vi "SNReport.vi"(6 "SN":string="1", 7 "Slot":T1, 8 "error in (no error)":errorcluster caption="错误输入（无错误）", 9 "字符串":string="测试报告\\条码\\", 10 "列首字符串":string[](array[string])=["ICCID", "IMSI", "AKEY", "ESN", "EVDO账号", "EVDO密码", "MDN", "MEID", "T-BOX-SN", "时间"]) -> (0 "error out":errorcluster caption="错误输出")   [LabVIEW 2013]
uses:
  SystemCode/SysControl/Slot.ctl
  <vilib>/addons/_office/_wordsub.llb/font.ctl
  <vilib>/Utility/NIReport.llb/NI_report.lvclass
  GlobalValue.vi
  <vilib>/addons/_office/excel.llb/Excel Easy Table (str).vi
  <vilib>/Utility/NIReport.llb/Append Text Table to Report (wrap).vi
  <vilib>/addons/_office/NI_ReportGenerationToolkit.lvlib
  <vilib>/Utility/NIReport.llb/Excel/NI_Excel.lvclass
panel:
  out "数组":string[][](array[string])
  in  "TestItem":string="BCM"
  # "产品名称\t序列号\t测试时间\t测试项目\t初始条件\t测试动作\t评价标准\t步骤 测试结果\t测试条件设置"
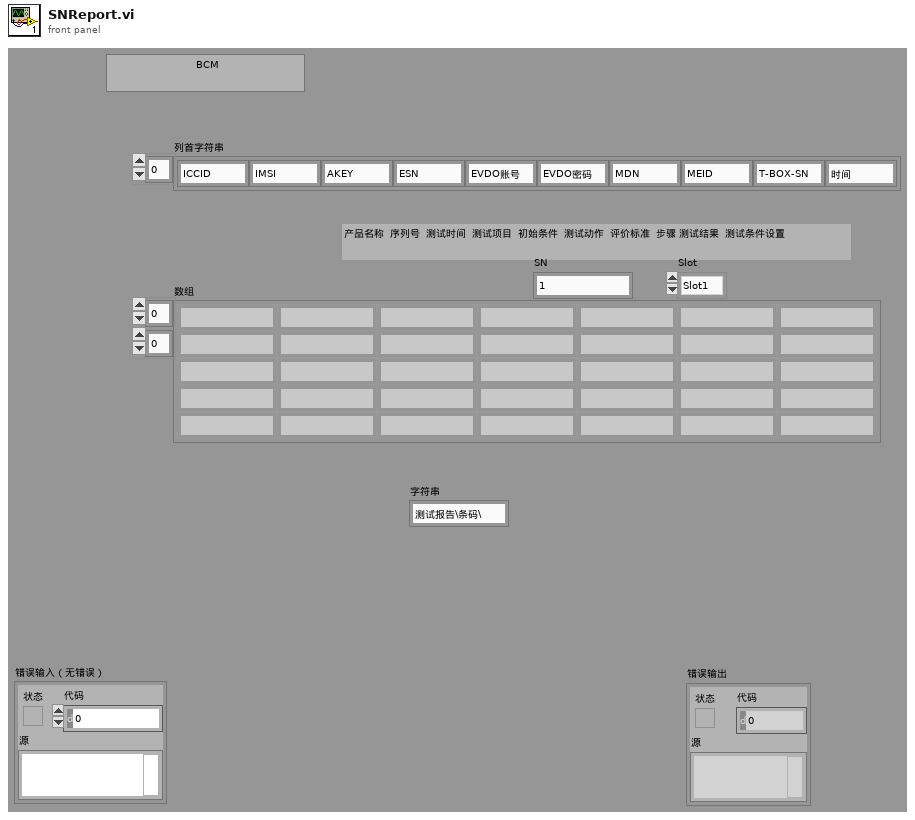
[diagram p1: front panel]
types:
  T1 = typedef "Slot.ctl" = enum16{"Slot1", "Slot2", "Slot3", "Slot4"}
  T2 = enum16{"open", "replace", "create", "open or create", "replace or create", "replace or create with confirmation"}
  T3 = typedef "font.ctl" = cluster{"font name":string, "font size":dbl, "bold":u16, "italic":u16, "underline":u16, "strike through":u16, "font color":u32}
  T4 = enum16{"maximized", "minimized", "normal", "no change"}
  T5 = enum16{"Standard Report", "HTML", "Word", "Excel"}
  T6 = cluster{"on/off":bool, "weight":i32, "color":u32}
  T7 = cluster{"position (Excel)":cluster{"row":i32, "column":i32}, "name (Excel)":string, "bookmark (Word)":string}
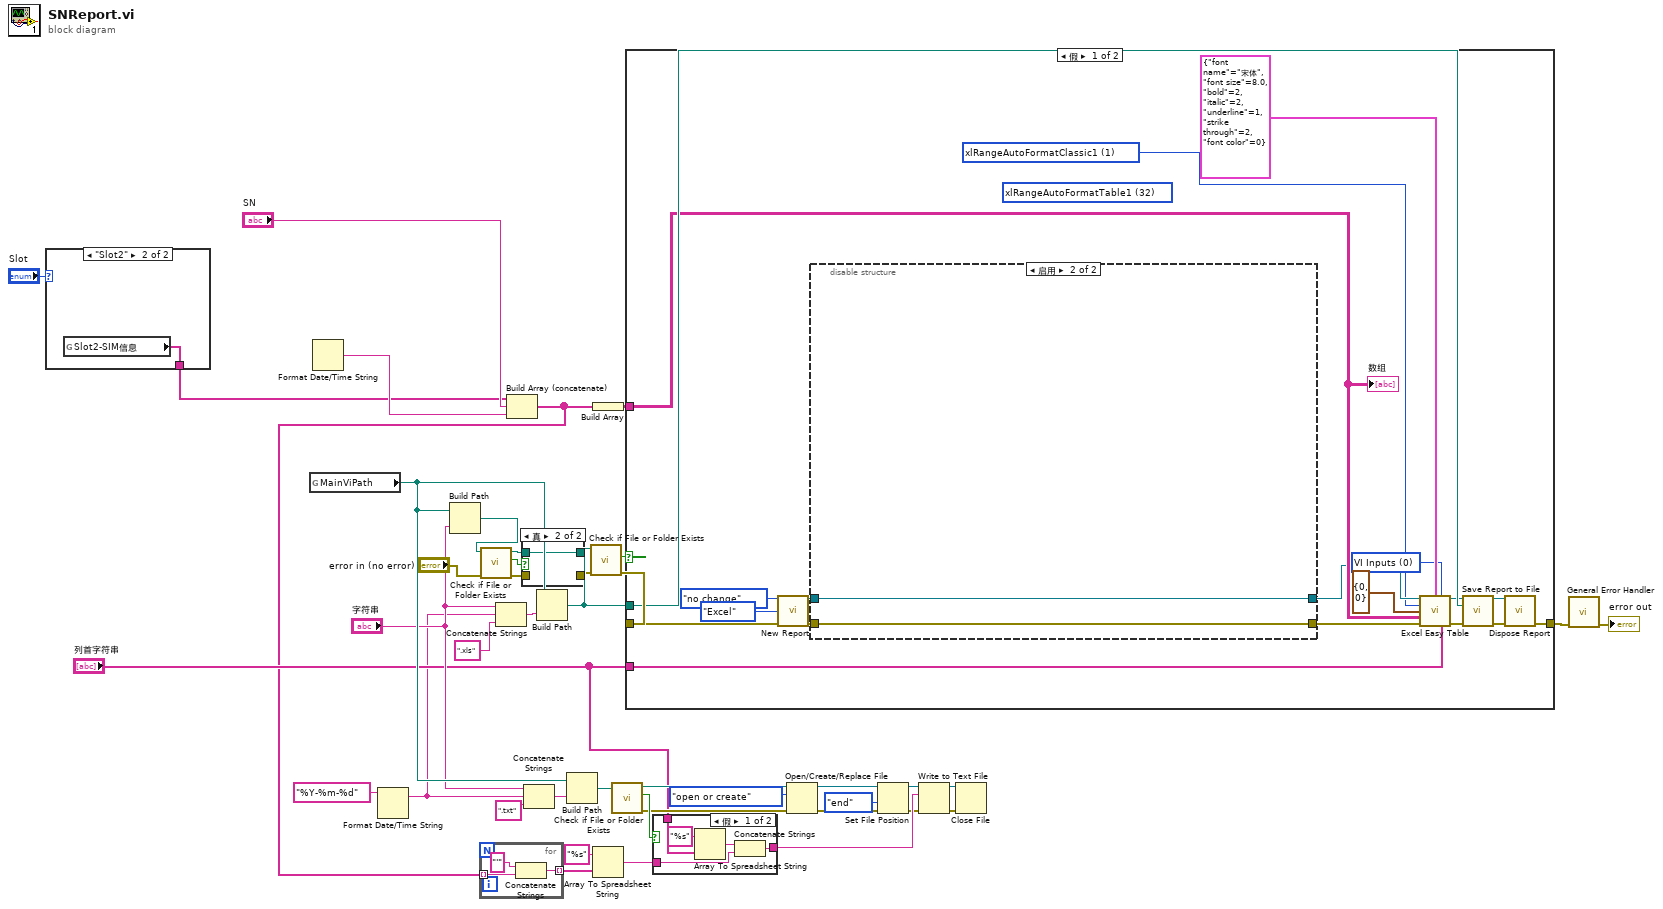
[diagram p0: block diagram]
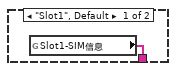
[diagram p3: hidden frame]
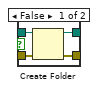
[diagram p4: hidden frame]
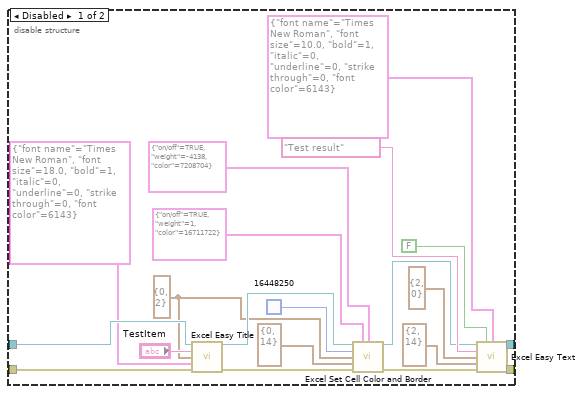
[diagram p5: hidden frame]
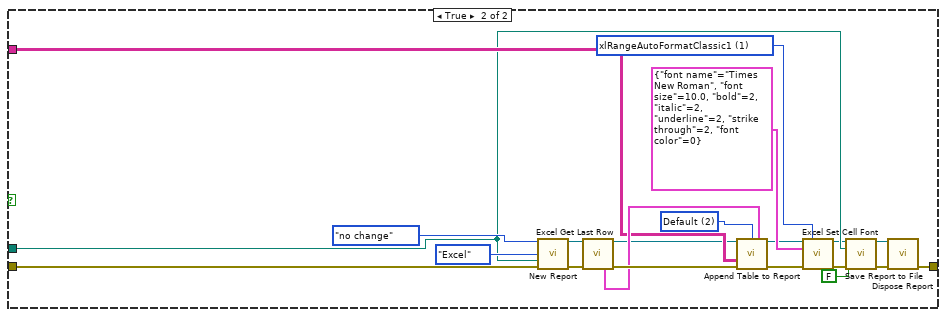
[diagram p6: hidden frame]
diagram:
  n1 = case shown="\"Slot2\"" "Slot" {
    tunnel: [w43 w44] -> w4
    frame "Slot1", Default {
      n2 = global read "GlobalValue.vi" "Slot1-SIM信息"() -> (w43:string[])
    }
    frame "Slot2" {
      n3 = global read "GlobalValue.vi" "Slot2-SIM信息"() -> (w44:string[])
    }
  }
  n4 = global read "GlobalValue.vi" "MainViPath"() -> (w7:path)
  n5 = Format Date/Time String() -> (date/time string=w26:string)  [unwired: 3 in]
  n6 = Format Date/Time String(time format string (%c)="%Y-%m-%d" ("时间格式字符串(%c)")) -> (date/time string=w1:string)  [unwired: 2 in]
  n7 = Build Path(base path=w7, name or relative path="字符串") -> (appended path=w33:path)
  n8 = call <vilib>:"Check if File or Folder Exists.vi"("error in (no error)"="error in (no error)", "path"=w33) -> ("error out"=w35:errorcluster, "file or folder exists?"=w34:bool, "dup path"=w36:path)  [unwired: 7 out]
  n9 = Concatenate Strings("字符串", w1, ".xls" ("连接的字符串")) -> (w38:string)
  n10 = Build Array (concatenate)(w4, "SN", w26) -> (w3:string[])
  n11 = for {
    tunnel: w3 -> [w47] mode=indexing
    tunnel: [w45] -> w20 mode=indexing
    n12 = Concatenate Strings("'" ("字符串"), w47) -> (w45:string)
  }
  n13 = case shown="真" w34 {
    tunnel: w36 -> [w51 w52]
    tunnel: [w50 _] -> w31
    tunnel: w35 -> [w49 _]
    tunnel: [w48 w52] -> _
    frame False {
      n14 = Create Folder(path (use dialog)=w51, error in=w49) -> (created path=w48:path, error out=w50:errorcluster)  [unwired: 2 out]
    }
    frame True {
    }
  }
  n15 = Concatenate Strings("字符串", w1, ".txt" ("连接的字符串")) -> (w17:string)
  n16 = Build Path(base path=w7, name or relative path=w38) -> (appended path=w42:path)
  n17 = Build Path(base path=w7, name or relative path=w17) -> (appended path=w16:path)
  n18 = call <vilib>:"Check if File or Folder Exists.vi"("error in (no error)"=w31, "path"=w42) -> ("error out"=w40:errorcluster, "file or folder exists?"=w39:bool)  [unwired: 8 out]
  n19 = Build Array(w3) -> (w28:string[][])
  n20 = Array To Spreadsheet String(array=w20, 3:"%s" ("格式字符串")) -> (spreadsheet string=w14:string)  [unwired: 1 in]
  n21 = call <vilib>:"Check if File or Folder Exists.vi"("path"=w16) -> ("error out"=w11:errorcluster, "file or folder exists?"=w15:bool, "dup path"=w12:path)  [unwired: 1 in, 7 out]
  n22 = case shown="假" w39 {
    tunnel: w40 -> [w70 w113]
    tunnel: w42 -> [w62 w106]
    tunnel: [w65 w112] -> w41
    tunnel: w28 -> [w61 w108]
    tunnel: "列首字符串" -> [w53 _]
    frame False {
      w54 = u16 0 items=["VI Inputs", "Font Dialog Box"] ("font settings source")
      w56 = 1 items=["xlRangeAutoFormat3DEffects1"=13, "xlRangeAutoFormat3DEffects2"=14, "xlRangeAutoFormatAccounting1"=4, "xlRangeAutoFormatAccounting2"=5, "xlRangeAutoFormatAccounting3"=6, "xlRangeAutoFormatAccounting4"=17, "xlRangeAutoFormatClassic1"=1, "xlRangeAutoFormatClassic2"=2, "xlRangeAutoFormatClassic3"=3, "xlRangeAutoFormatColor1"=7, "xlRangeAutoFormatColor2"=8, "xlRangeAutoFormatColor3"=9, "xlRangeAutoFormatList1"=10, "xlRangeAutoFormatList2"=11, "xlRangeAutoFormatList3"=12, "xlRangeAutoFormatLocalFormat1"=15, "xlRangeAutoFormatLocalFormat2"=16, "xlRangeAutoFormatLocalFormat3"=19, "xlRangeAutoFormatLocalFormat4"=20, "xlRangeAutoFormatReport1"=21, "xlRangeAutoFormatReport2"=22, "xlRangeAutoFormatReport3"=23, "xlRangeAutoFormatReport4"=24, "xlRangeAutoFormatReport5"=25, "xlRangeAutoFormatReport6"=26, "xlRangeAutoFormatReport7"=27, "xlRangeAutoFormatReport8"=28, "xlRangeAutoFormatReport9"=29, "xlRangeAutoFormatReport10"=30, "xlRangeAutoFormatClassicPivotTable"=31, "xlRangeAutoFormatTable1"=32, "xlRangeAutoFormatTable2"=33, "xlRangeAutoFormatTable3"=34, "xlRangeAutoFormatTable4"=35, "xlRangeAutoFormatTable5"=36, "xlRangeAutoFormatTable6"=37, "xlRangeAutoFormatTable7"=38, "xlRangeAutoFormatTable8"=39, "xlRangeAutoFormatTable9"=40, "xlRangeAutoFormatTable10"=41, "xlRangeAutoFormatPTNone"=42, "xlRangeAutoFormatNone"=-4142, "xlRangeAutoFormatSimple"=-4154] ("auto format")
      (unwired) 32 items=["xlRangeAutoFormat3DEffects1"=13, "xlRangeAutoFormat3DEffects2"=14, "xlRangeAutoFormatAccounting1"=4, "xlRangeAutoFormatAccounting2"=5, "xlRangeAutoFormatAccounting3"=6, "xlRangeAutoFormatAccounting4"=17, "xlRangeAutoFormatClassic1"=1, "xlRangeAutoFormatClassic2"=2, "xlRangeAutoFormatClassic3"=3, "xlRangeAutoFormatColor1"=7, "xlRangeAutoFormatColor2"=8, "xlRangeAutoFormatColor3"=9, "xlRangeAutoFormatList1"=10, "xlRangeAutoFormatList2"=11, "xlRangeAutoFormatList3"=12, "xlRangeAutoFormatLocalFormat1"=15, "xlRangeAutoFormatLocalFormat2"=16, "xlRangeAutoFormatLocalFormat3"=19, "xlRangeAutoFormatLocalFormat4"=20, "xlRangeAutoFormatReport1"=21, "xlRangeAutoFormatReport2"=22, "xlRangeAutoFormatReport3"=23, "xlRangeAutoFormatReport4"=24, "xlRangeAutoFormatReport5"=25, "xlRangeAutoFormatReport6"=26, "xlRangeAutoFormatReport7"=27, "xlRangeAutoFormatReport8"=28, "xlRangeAutoFormatReport9"=29, "xlRangeAutoFormatReport10"=30, "xlRangeAutoFormatClassicPivotTable"=31, "xlRangeAutoFormatTable1"=32, "xlRangeAutoFormatTable2"=33, "xlRangeAutoFormatTable3"=34, "xlRangeAutoFormatTable4"=35, "xlRangeAutoFormatTable5"=36, "xlRangeAutoFormatTable6"=37, "xlRangeAutoFormatTable7"=38, "xlRangeAutoFormatTable8"=39, "xlRangeAutoFormatTable9"=40, "xlRangeAutoFormatTable10"=41, "xlRangeAutoFormatPTNone"=42, "xlRangeAutoFormatNone"=-4142, "xlRangeAutoFormatSimple"=-4154] ("auto format")
      n23 = call <vilib>:"New Report.vi"("window state (normal)"=T4."no change", "report type"=T5."Excel", "error in (no error)"=w70) -> ("report out"=w66:refnum<class "NI_report.lvclass">, "error out"=w67:errorcluster)  [unwired: 3 in, 8 out]
      n24 = disable-structure shown="启用" {
        disable-tunnel: w67 -> [w90 w93]
        disable-tunnel: w66 -> [w89 w92]
        disable-tunnel: [w73 w92] -> w59
        disable-tunnel: [w72 w93] -> w58
        frame Disabled {
          w78 = cluster{"row":i32, "column":i32} {"row"=0, "column"=2} ("start")
          n25 = call <vilib>:"Excel Easy Title.vi"("report in"=w89, "title"="TestItem", "start (0, 0)"=w78, "font"=T3 {"font name"="Times New Roman", "font size"=18.0, "bold"=1, "italic"=0, "underline"=0, "strike through"=0, "font color"=6143}, "error in (no error)"=w90) -> ("report out"=w82:refnum<class "NI_report.lvclass">, "error out"=w81:errorcluster)  [unwired: 8 in, 1 out]
          n26 = call <vilib>:"Excel Set Cell Color and Border.vi"("report in"=w82, "inside border"=T6 {"on/off"=TRUE, "weight"=1, "color"=16711722}, "outside border"=T6 {"on/off"=TRUE, "weight"=-4138, "color"=7208704} ("inside border"), "background color (w)"=u32 16448250 ("color"), "start (-1, -1)"=w78, "end (-1, -1)"=cluster{"row":i32, "column":i32} {"row"=0, "column"=14} ("start"), "error in (no error)"=w81) -> ("report out"=w75:refnum<class "NI_report.lvclass">, "error out"=w74:errorcluster)  [unwired: 7 in]
          n27 = call <vilib>:"Excel Easy Text.vi"("report in"=w75, "border? (F)"=FALSE, "font"=T3 {"font name"="Times New Roman", "font size"=10.0, "bold"=1, "italic"=0, "underline"=0, "strike through"=0, "font color"=6143}, "text"="Test result" ("font name"), "start (-1, -1)"=cluster{"row":i32, "column":i32} {"row"=2, "column"=0} ("start"), "end (-1, -1)"=cluster{"row":i32, "column":i32} {"row"=2, "column"=14} ("start"), "error in (no error)"=w74) -> ("report out"=w73:refnum<class "NI_report.lvclass">, "error out"=w72:errorcluster)  [unwired: 4 in, 3 out]
        }
        frame Enabled {
        }
      }
      n28 = call-poly <vilib>:"Excel Easy Table.vi"("report in"=w59, "font"=T3 {"font name"="宋体", "font size"=8.0, "bold"=2, "italic"=2, "underline"=1, "strike through"=2, "font color"=0}, "font settings source"=w54, "auto format (none)"=w56, "start (0, 0)"=cluster{"row":i32, "column":i32} {"row"=0, "column"=0} ("position"), "text data"=w61, "error in (no error)"=w58, "column headers"=w53) -> ("report out"=w57:refnum<class "NI_report.lvclass">, "error out"=w64:errorcluster)  [unwired: 3 in, 3 out]
      n29 = call-dynamic "Save Report to File.vi"("report in"=w57, "report file path"=w62, "error in (no error)"=w64) -> ("report out"=w63:refnum<class "NI_report.lvclass">, "error out"=w60:errorcluster)  [unwired: 2 in, 9 out]
      n30 = call-dynamic "Dispose Report.vi"("report in"=w63, "error in (no error)"=w60) -> ("error out"=w65:errorcluster)  [unwired: 13 in]
      "数组" <- w61
    }
    frame True {
      w100 = 1 items=["xlRangeAutoFormat3DEffects1"=13, "xlRangeAutoFormat3DEffects2"=14, "xlRangeAutoFormatAccounting1"=4, "xlRangeAutoFormatAccounting2"=5, "xlRangeAutoFormatAccounting3"=6, "xlRangeAutoFormatAccounting4"=17, "xlRangeAutoFormatClassic1"=1, "xlRangeAutoFormatClassic2"=2, "xlRangeAutoFormatClassic3"=3, "xlRangeAutoFormatColor1"=7, "xlRangeAutoFormatColor2"=8, "xlRangeAutoFormatColor3"=9, "xlRangeAutoFormatList1"=10, "xlRangeAutoFormatList2"=11, "xlRangeAutoFormatList3"=12, "xlRangeAutoFormatLocalFormat1"=15, "xlRangeAutoFormatLocalFormat2"=16, "xlRangeAutoFormatLocalFormat3"=19, "xlRangeAutoFormatLocalFormat4"=20, "xlRangeAutoFormatReport1"=21, "xlRangeAutoFormatReport2"=22, "xlRangeAutoFormatReport3"=23, "xlRangeAutoFormatReport4"=24, "xlRangeAutoFormatReport5"=25, "xlRangeAutoFormatReport6"=26, "xlRangeAutoFormatReport7"=27, "xlRangeAutoFormatReport8"=28, "xlRangeAutoFormatReport9"=29, "xlRangeAutoFormatReport10"=30, "xlRangeAutoFormatClassicPivotTable"=31, "xlRangeAutoFormatTable1"=32, "xlRangeAutoFormatTable2"=33, "xlRangeAutoFormatTable3"=34, "xlRangeAutoFormatTable4"=35, "xlRangeAutoFormatTable5"=36, "xlRangeAutoFormatTable6"=37, "xlRangeAutoFormatTable7"=38, "xlRangeAutoFormatTable8"=39, "xlRangeAutoFormatTable9"=40, "xlRangeAutoFormatTable10"=41, "xlRangeAutoFormatPTNone"=42, "xlRangeAutoFormatNone"=-4142, "xlRangeAutoFormatSimple"=-4154] ("auto format")
      w102 = u16 2 items=["US", "Metric", "Default"] ("measurement system")
      n31 = call <vilib>:"New Report.vi"("window state (normal)"=T4."no change", "report type"=T5."Excel", "template (empty)"=w106, "error in (no error)"=w113) -> ("report out"=w103:refnum<class "NI_report.lvclass">, "error out"=w111:errorcluster)  [unwired: 2 in, 8 out]
      n32 = call <vilib>:"Excel Get Last Row.vi"("report in"=w103, "error in (no error)"=w111) -> ("report out"=w99:refnum<class "NI_report.lvclass">, "MS Office parameters out"=w109:T7, "error out"=w110:errorcluster)  [unwired: 1 in, 10 out]
      n33 = call-poly <vilib>:"Append Table to Report.vi"("report in"=w99, "measurement system"=w102, "MS Office parameters"=w109, "text data"=w108, "error in (no error)"=w110) -> ("report out"=w96:refnum<class "NI_report.lvclass">, "error out"=w98:errorcluster)  [unwired: 5 in, 4 out]
      n34 = call <vilib>:"Excel Set Cell Font.vi"("report in"=w96, "auto format"=w100, "font"=T3 {"font name"="Times New Roman", "font size"=10.0, "bold"=2, "italic"=2, "underline"=2, "strike through"=2, "font color"=0}, "error in (no error)"=w98) -> ("report out"=w95:refnum<class "NI_report.lvclass">, "error out"=w97:errorcluster)  [unwired: 10 in]
      n35 = call-dynamic "Save Report to File.vi"("report in"=w95, "report file path"=w106, "prompt to replace? (F)"=FALSE, "error in (no error)"=w97) -> ("report out"=w104:refnum<class "NI_report.lvclass">, "error out"=w105:errorcluster)  [unwired: 1 in, 9 out]
      n36 = call-dynamic "Dispose Report.vi"("report in"=w104, "error in (no error)"=w105) -> ("error out"=w112:errorcluster)  [unwired: 3 in, 10 out]
    }
  }
  n37 = case shown="假" w15 {
    tunnel: "列首字符串" -> [w117 _]
    tunnel: w14 -> [w116 w120]
    tunnel: [w115 w120] -> w13
    frame False {
      n38 = Array To Spreadsheet String(array=w117, 3:"%s" ("格式字符串")) -> (spreadsheet string=w119:string)  [unwired: 1 in]
      n39 = Concatenate Strings(w119, w116) -> (w115:string)
    }
    frame True {
    }
  }
  n40 = Open/Create/Replace File(file path (use dialog)=w12, error in=w11, operation (0:open)=T2."open or create" ("操作(0:open)")) -> (refnum out=w24:refnum<file>, error out=w10:errorcluster)  [unwired: 3 in, 1 out]
  n41 = Set File Position(refnum=w24, from (0:start)=enum16{"start", "end", "current"}."end" ("自（0:起始）"), error in=w10) -> (refnum out=w22:refnum<file>, error out=w9:errorcluster)  [unwired: 1 in]
  n42 = Write to Text File(file (use dialog)=w22, text=w13, error in=w9) -> (refnum out=w21:refnum<file>, error out=w8:errorcluster)  [unwired: 1 in, 1 out]
  n43 = Close File(refnum=w21, error in=w8) -> ()  [unwired: 2 out]
  n44 = call <vilib>:"General Error Handler.vi"("error in (no error)"=w41) -> ("error out"=→"error out":errorcluster)  [unwired: 10 in, 4 out]
